vi "Basic ITC-IL.vi"(4 "Interval between messages (ms)":i16=10, 5 "ISOBUS address":T4=-1, 6 "error in (no error)":errorcluster, 7 "Device_Present?":bool[](array[boolean]), 8 "Ch_type_index":i32[](array[numeric]), 9 "Merc_ref_Array":T1[](array[typedef])) -> (0 "error out":errorcluster, 2 "Ch Info":T5(array[cluster]))   [LabVIEW 2013, in "Mercury iXX.lvlib"]
uses:
  Mercury iXX.lvlib
  Public/Libraries/Temperature/Signals/Read/Temperature (Read).vi
  Public/Libraries/Temperature.lvlib
  Public/Libraries/Level Meter/Signals/Read/Probe Level Helium (Read).vi
  Public/Libraries/Level Meter.lvlib
  Public/Libraries/Level Meter/Signals/Read/Probe Level Nitrogen (Read).vi
  Public/Controls/Comms Transport Layer.ctl
  Private/Controls/Query Dynamic Reference.ctl
  Public/Controls/Mercury Reference.ctl
  Public/Libraries/Heater/Signals/Read/Voltage (Read).vi
  Public/Libraries/Heater.lvlib
  Public/Libraries/Heater/Signals/Read/Current (Read).vi
  Public/Libraries/Heater/Signals/Read/Power (Read).vi
  Public/Libraries/Temperature/Signals/Read/Voltage (Read).vi
  Public/Libraries/Temperature/Signals/Read/Resistance (Read).vi
  Public/Libraries/Auxiliary/Signals/Read/Percent Open (Read).vi
  Public/Libraries/Auxiliary.lvlib
  Public/Libraries/Auxiliary/Signals/Read/Position (Read).vi
  Public/Libraries/Level Meter/Signals/Read/Probe Resistance Helium (Read).vi
  Public/Libraries/Level Meter/Signals/Read/Probe Frequency Nitrogen (Read).vi
  Public/Libraries/Pressure/Signals/Read/Pressure (Read).vi
  Public/Libraries/Pressure.lvlib
  Public/Libraries/Pressure/Signals/Read/Voltage (Read).vi
  Public/Libraries/Pressure/Signals/Read/Current (Read).vi
  Public/Libraries/Pressure/Signals/Read/Power (Read).vi
  Public/Controls/ISOBus Address.ctl
panel:
  in  "Tab Control":enum32{"Link Panel", "Front_Panel", "Error"}(tab)
  # "MB0\nMB1\nDB1\nDB2\nDB3\nDB4\nDB5\nDB6\nDB7\nDB8"
  # "Switch Controls"
  # "MercuryiTC-VI"
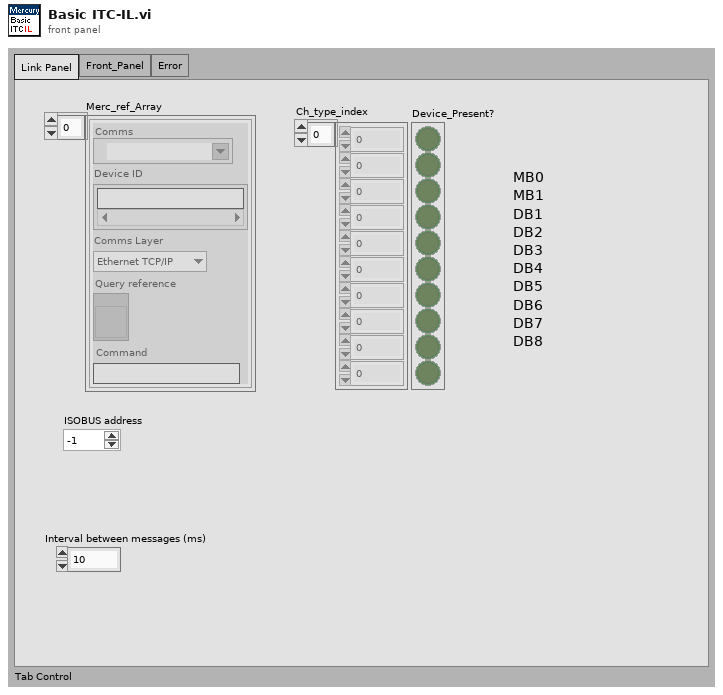
[diagram p1: front panel]
types:
  T1 = typedef "Mercury iXX.lvlib/Mercury Reference.ctl" = cluster{"Comms":refnum<visa-resource-name>, "Device ID":string[], "Comms Layer":T2, "Command":string, "Query reference":T3}
  T2 = typedef "Mercury iXX.lvlib/Comms Transport Layer.ctl" = enum16{"Ethernet TCP/IP", "USB", "ISOBus - RS-232", "GPIB"}
  T3 = typedef "Mercury iXX.lvlib/Query Dynamic Reference.ctl" = refnum<vi>
  T4 = typedef "Mercury iXX.lvlib/ISOBus Address.ctl" = i32
  T5 = cluster{"Data":string[], "Label":string[], "Units":string[], "Channel":string, "Type":string}[]
  T6 = cluster{"Data":string[], "Label":string[], "Units":string[], "Channel":string, "Type":string}
  T7 = typedef "Mercury iXX.lvlib/Unit String.ctl" = string
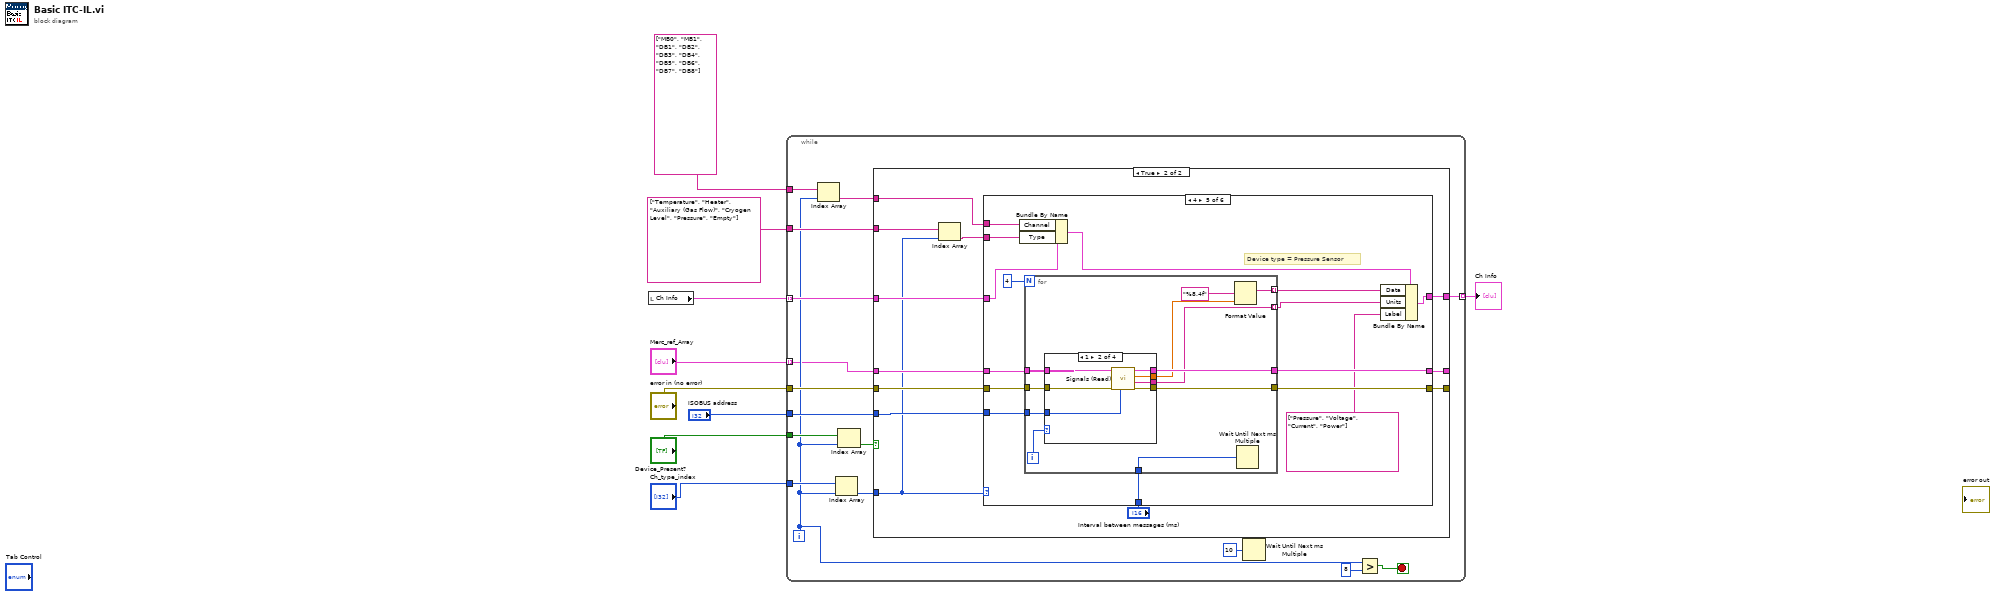
[diagram p0: block diagram]
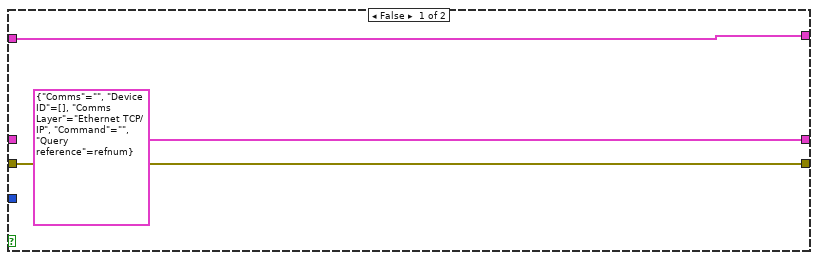
[diagram p2: hidden frame]
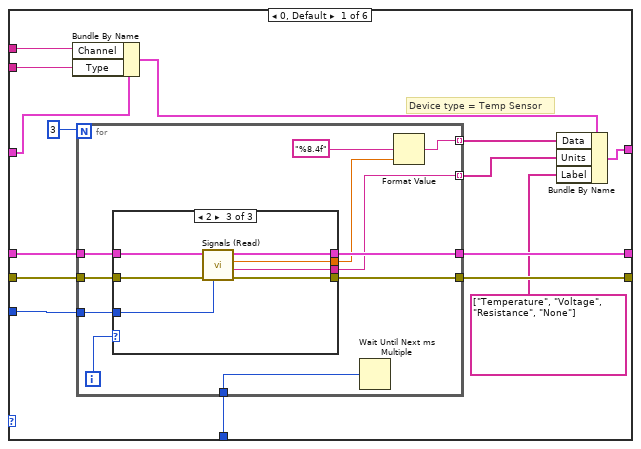
[diagram p3: hidden frame]
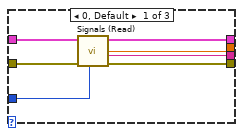
[diagram p4: hidden frame]
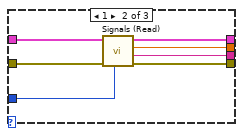
[diagram p5: hidden frame]
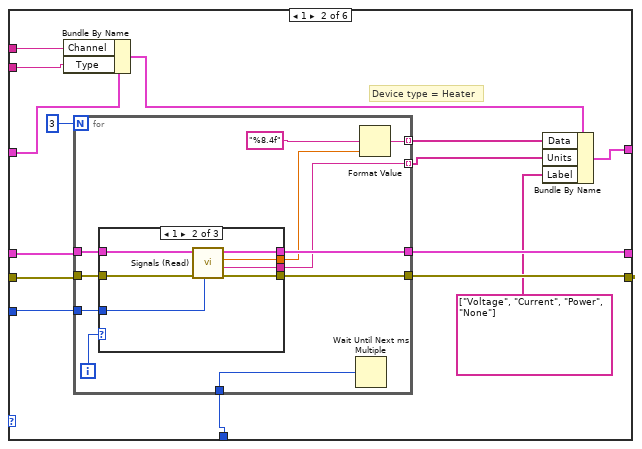
[diagram p6: hidden frame]
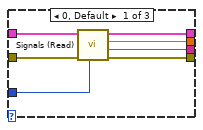
[diagram p7: hidden frame]
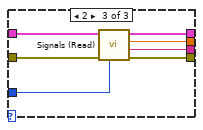
[diagram p8: hidden frame]
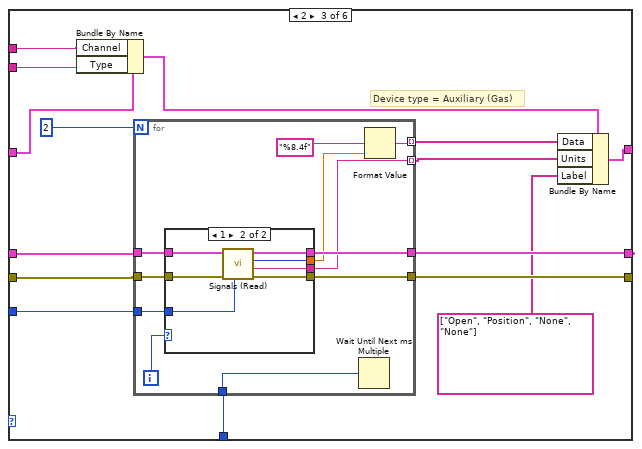
[diagram p9: hidden frame]
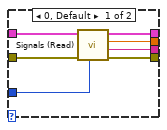
[diagram p10: hidden frame]
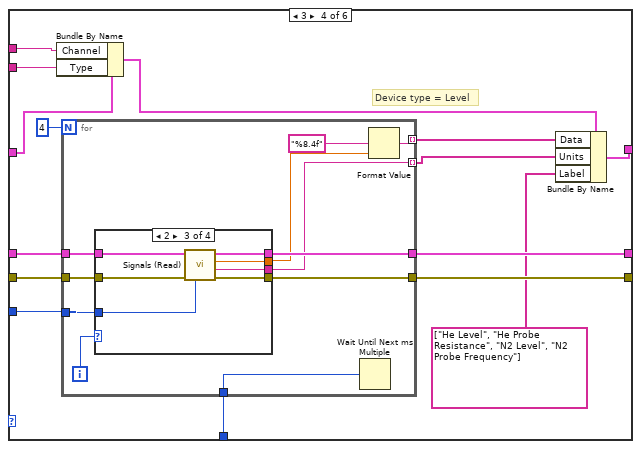
[diagram p11: hidden frame]
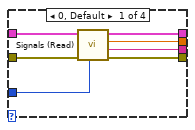
[diagram p12: hidden frame]
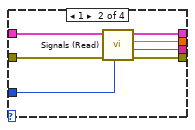
[diagram p13: hidden frame]
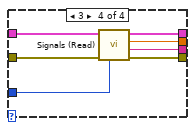
[diagram p14: hidden frame]
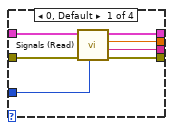
[diagram p15: hidden frame]
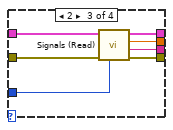
[diagram p16: hidden frame]
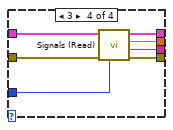
[diagram p17: hidden frame]
diagram:
  n1 = local read "Ch Info"() -> (w9:T5)
  n2 = while {
    tunnel: "Ch_type_index" -> [w25]
    tunnel: "Device_Present?" -> [w24]
    tunnel: "Merc_ref_Array" -> [w10] mode=indexing
    tunnel: "error in (no error)" -> [w21]
    tunnel: "ISOBUS address" -> [w20]
    tunnel: w9 -> [w19] mode=indexing
    tunnel: [w18] -> w3 mode=indexing
    tunnel: string[] ["Temperature", "Heater", "Auxiliary (Gas Flow)", "Cryogen Level", "Pressure", "Empty"] -> [w14]
    tunnel: string[] ["MB0", "MB1", "DB1", "DB2", "DB3", "DB4", "DB5", "DB6", "DB7", "DB8"] -> [w13]
    i -> [w12]
    stop <- w17 stop-if-true
    n3 = Index Array(array=w13, index=w12) -> (element=w11:string)
    n4 = Index Array(array=w25, index=w12) -> (element=w22:i32)
    n5 = Index Array(array=w24, index=w12) -> (element=w23:bool)
    n6 = case shown="True" w23 {
      tunnel: w10 -> [_ w40]
      tunnel: w22 -> [_ w31]
      tunnel: w21 -> [w27 w39]
      tunnel: w20 -> [_ w38]
      tunnel: [w27 w37] -> _
      tunnel: [T1 {"Comms"="", "Device ID"=[], "Comms Layer"=enum."Ethernet TCP/IP", "Command"="", "Query reference"=refnum} ("MB1.T1_Ref") w36] -> _
      tunnel: w19 -> [w26 w34]
      tunnel: [w26 w33] -> w18
      tunnel: w14 -> [_ w32]
      tunnel: w11 -> [_ w29]
      frame False {
      }
      frame True {
        n7 = Index Array(array=w32, index=w31) -> (element=w30:string)
        n8 = case shown="4" w31 {
          tunnel: w40 -> [w55 w102 w149 w189 w243 w285]
          tunnel: w39 -> [w54 w101 w148 w188 w242 w284]
          tunnel: w38 -> [w52 w100 w147 w187 w241 _]
          tunnel: [w51 w98 w145 w185 w239 w285] -> w36
          tunnel: [w50 w97 w144 w184 w238 w284] -> w37
          tunnel: "Interval between messages (ms)" -> [w53 w99 w146 w186 w240 _]
          tunnel: w34 -> [w41 w89 w138 w176 w230 w283]
          tunnel: [w48 w95 w142 w182 w236 w283] -> w33
          tunnel: w30 -> [w44 w90 w136 w177 w231 _]
          tunnel: w29 -> [w43 w91 w137 w178 w232 _]
          frame 0, Default {
            # "Device type = Temp Sensor"
            n9 = Bundle By Name(cluster=w41, "Channel"=w43, "Type"=w44) -> (w42:T6)
            n10 = for {
              N: 3 -> [_]
              tunnel: w55 -> [w65]
              tunnel: w54 -> [w64]
              tunnel: w53 -> [w63]
              tunnel: w52 -> [w62]
              tunnel: [w61] -> w51
              tunnel: [w60] -> w50
              tunnel: [w58] -> w47 mode=indexing
              tunnel: [w56] -> w45 mode=indexing
              i -> [w66]
              n11 = case shown="2" w66 {
                tunnel: w65 -> [w73 w80 w86]
                tunnel: w64 -> [w72 w79 w85]
                tunnel: w62 -> [w71 w78 w87]
                tunnel: [w70 w77 w84] -> w61
                tunnel: [w69 w76 w83] -> w60
                tunnel: [w68 w75 w82] -> w59
                tunnel: [w67 w74 w81] -> w56
                frame 0, Default {
                  n12 = call-poly "Signals (Read).vi"("ISOBUS address"=w71, "error in"=w72, "Mercury Reference In"=w73) -> ("error out"=w69:errorcluster, "Unit"=w67:T7, "Temperature"=w68:dbl, "Mercury Reference Out"=w70:T1)  [unwired: 4 in, 1 out]
                }
                frame 1 {
                  n13 = call-poly "Signals (Read).vi"("ISOBUS address"=w78, "error in"=w79, "Mercury Reference In"=w80) -> ("error out"=w76:errorcluster, "Unit"=w74:T7, "Voltage"=w75:dbl, "Mercury Reference Out"=w77:T1)  [unwired: 4 in, 1 out]
                }
                frame 2 {
                  n14 = call-poly "Signals (Read).vi"("ISOBUS address"=w87, "error in"=w85, "Mercury Reference In"=w86) -> ("error out"=w83:errorcluster, "Unit"=w81:T7, "Resistance"=w82:dbl, "Mercury Reference Out"=w84:T1)  [unwired: 4 in, 1 out]
                }
              }
              n15 = Wait Until Next ms Multiple(millisecond multiple=w63) -> ()  [unwired: 1 out]
              n16 = Format Value(format string="%8.4f", value (0)=w59) -> (output string=w58:string)  [unwired: 1 in]
            }
            n17 = Bundle By Name(cluster=w42, "Data"=w47, "Units"=w45, "Label"=string[] ["Temperature", "Voltage", "Resistance", "None"]) -> (w48:T6)
          }
          frame 1 {
            # "Device type = Heater"
            n18 = Bundle By Name(cluster=w89, "Channel"=w91, "Type"=w90) -> (w88:T6)
            n19 = for {
              N: 3 -> [_]
              tunnel: w102 -> [w112]
              tunnel: w101 -> [w111]
              tunnel: w99 -> [w110]
              tunnel: w100 -> [w109]
              tunnel: [w108] -> w98
              tunnel: [w107] -> w97
              tunnel: [w105] -> w94 mode=indexing
              tunnel: [w103] -> w92 mode=indexing
              i -> [w113]
              n20 = case shown="1" w113 {
                tunnel: w112 -> [w120 w127 w133]
                tunnel: w111 -> [w119 w126 w132]
                tunnel: w109 -> [w118 w125 w134]
                tunnel: [w117 w124 w131] -> w108
                tunnel: [w116 w123 w130] -> w107
                tunnel: [w115 w122 w129] -> w106
                tunnel: [w114 w121 w128] -> w103
                frame 0, Default {
                  n21 = call-poly "Signals (Read).vi"("ISOBUS address"=w118, "error in"=w119, "Mercury Reference In"=w120) -> ("error out"=w116:errorcluster, "Unit"=w114:T7, "Voltage"=w115:dbl, "Mercury Reference Out"=w117:T1)  [unwired: 4 in, 1 out]
                }
                frame 1 {
                  n22 = call-poly "Signals (Read).vi"("ISOBUS address"=w125, "error in"=w126, "Mercury Reference In"=w127) -> ("error out"=w123:errorcluster, "Unit"=w121:T7, "Current"=w122:dbl, "Mercury Reference Out"=w124:T1)  [unwired: 4 in, 1 out]
                }
                frame 2 {
                  n23 = call-poly "Signals (Read).vi"("ISOBUS address"=w134, "error in"=w132, "Mercury Reference In"=w133) -> ("error out"=w130:errorcluster, "Unit"=w128:T7, "Power"=w129:dbl, "Mercury Reference Out"=w131:T1)  [unwired: 4 in, 1 out]
                }
              }
              n24 = Wait Until Next ms Multiple(millisecond multiple=w110) -> ()  [unwired: 1 out]
              n25 = Format Value(format string="%8.4f", value (0)=w106) -> (output string=w105:string)  [unwired: 1 in]
            }
            n26 = Bundle By Name(cluster=w88, "Data"=w94, "Units"=w92, "Label"=string[] ["Voltage", "Current", "Power", "None"]) -> (w95:T6)
          }
          frame 2 {
            # "Device type = Auxiliary (Gas)"
            n27 = Bundle By Name(cluster=w138, "Channel"=w137, "Type"=w136) -> (w135:T6)
            n28 = for {
              N: 2 -> [_]
              tunnel: w149 -> [w159]
              tunnel: w148 -> [w158]
              tunnel: w146 -> [w157]
              tunnel: w147 -> [w156]
              tunnel: [w155] -> w145
              tunnel: [w154] -> w144
              tunnel: [w151] -> w141 mode=indexing
              tunnel: [w150] -> w139 mode=indexing
              i -> [w160]
              n29 = case shown="1" w160 {
                tunnel: w159 -> [w167 w174]
                tunnel: w158 -> [w166 w173]
                tunnel: w156 -> [w165 w172]
                tunnel: [w164 w171] -> w155
                tunnel: [w163 w170] -> w154
                tunnel: [w162 w169] -> w152
                tunnel: [w161 w168] -> w150
                frame 0, Default {
                  n30 = call-poly "Signals (Read).vi"("ISOBUS address"=w165, "error in"=w166, "Mercury Reference In"=w167) -> ("error out"=w163:errorcluster, "Unit"=w161:T7, "% Open"=w162:dbl, "Mercury Reference Out"=w164:T1)  [unwired: 4 in, 1 out]
                }
                frame 1 {
                  n31 = call-poly "Signals (Read).vi"("ISOBUS address"=w172, "error in"=w173, "Mercury Reference In"=w174) -> ("error out"=w170:errorcluster, "Unit"=w168:T7, "Position"=w169:u32, "Mercury Reference Out"=w171:T1)  [unwired: 4 in, 1 out]
                }
              }
              n32 = Wait Until Next ms Multiple(millisecond multiple=w157) -> ()  [unwired: 1 out]
              n33 = Format Value(format string="%8.4f", value (0)=w152) -> (output string=w151:string)  [unwired: 1 in]
            }
            n34 = Bundle By Name(cluster=w135, "Data"=w141, "Units"=w139, "Label"=string[] ["Open", "Position", "None", "None"]) -> (w142:T6)
          }
          frame 3 {
            # "Device type = Level"
            n35 = Bundle By Name(cluster=w176, "Channel"=w178, "Type"=w177) -> (w175:T6)
            n36 = for {
              N: 4 -> [_]
              tunnel: w189 -> [w199]
              tunnel: w188 -> [w198]
              tunnel: w186 -> [w197]
              tunnel: w187 -> [w196]
              tunnel: [w195] -> w185
              tunnel: [w194] -> w184
              tunnel: [w191] -> w181 mode=indexing
              tunnel: [w190] -> w179 mode=indexing
              i -> [w200]
              n37 = case shown="2" w200 {
                tunnel: w199 -> [w207 w214 w220 w227]
                tunnel: w198 -> [w206 w213 w219 w226]
                tunnel: w196 -> [w205 w212 w221 w228]
                tunnel: [w204 w211 w218 w225] -> w195
                tunnel: [w203 w210 w217 w224] -> w194
                tunnel: [w202 w209 w216 w223] -> w192
                tunnel: [w201 w208 w215 w222] -> w190
                frame 0, Default {
                  n38 = call-poly "Signals (Read).vi"("ISOBUS address"=w205, "error in"=w206, "Mercury Reference In"=w207) -> ("error out"=w203:errorcluster, "Unit"=w201:T7, "Level"=w202:dbl, "Mercury Reference Out"=w204:T1)  [unwired: 4 in, 1 out]
                }
                frame 1 {
                  n39 = call-poly "Signals (Read).vi"("ISOBUS address"=w212, "error in"=w213, "Mercury Reference In"=w214) -> ("error out"=w210:errorcluster, "Unit"=w208:T7, "Resistance"=w209:dbl, "Mercury Reference Out"=w211:T1)  [unwired: 4 in, 1 out]
                }
                frame 2 {
                  n40 = call-poly "Signals (Read).vi"("ISOBUS address"=w221, "error in"=w219, "Mercury Reference In"=w220) -> ("error out"=w217:errorcluster, "Unit"=w215:T7, "Level"=w216:dbl, "Mercury Reference Out"=w218:T1)  [unwired: 4 in, 1 out]
                }
                frame 3 {
                  n41 = call-poly "Signals (Read).vi"("ISOBUS address"=w228, "error in"=w226, "Mercury Reference In"=w227) -> ("error out"=w224:errorcluster, "Unit"=w222:T7, "Freq"=w223:dbl, "Mercury Reference Out"=w225:T1)  [unwired: 4 in, 1 out]
                }
              }
              n42 = Wait Until Next ms Multiple(millisecond multiple=w197) -> ()  [unwired: 1 out]
              n43 = Format Value(format string="%8.4f", value (0)=w192) -> (output string=w191:string)  [unwired: 1 in]
            }
            n44 = Bundle By Name(cluster=w175, "Data"=w181, "Units"=w179, "Label"=string[] ["He Level", "He Probe Resistance", "N2 Level", "N2 Probe Frequency"]) -> (w182:T6)
          }
          frame 4 {
            # "Device type = Pressure Sensor"
            n45 = Bundle By Name(cluster=w230, "Channel"=w232, "Type"=w231) -> (w229:T6)
            n46 = for {
              N: 4 -> [_]
              tunnel: w243 -> [w253]
              tunnel: w242 -> [w252]
              tunnel: w240 -> [w251]
              tunnel: w241 -> [w250]
              tunnel: [w249] -> w239
              tunnel: [w248] -> w238
              tunnel: [w245] -> w235 mode=indexing
              tunnel: [w244] -> w233 mode=indexing
              i -> [w254]
              n47 = case shown="1" w254 {
                tunnel: w253 -> [w261 w268 w274 w281]
                tunnel: w252 -> [w260 w267 w273 w280]
                tunnel: w250 -> [w259 w266 w275 w282]
                tunnel: [w258 w265 w272 w279] -> w249
                tunnel: [w257 w264 w271 w278] -> w248
                tunnel: [w256 w263 w270 w277] -> w247
                tunnel: [w255 w262 w269 w276] -> w244
                frame 0, Default {
                  n48 = call-poly "Signals (Read).vi"("ISOBUS address"=w259, "error in"=w260, "Mercury Reference In"=w261) -> ("error out"=w257:errorcluster, "Unit"=w255:T7, "Temperature"=w256:dbl, "Mercury Reference Out"=w258:T1)  [unwired: 4 in, 1 out]
                }
                frame 1 {
                  n49 = call-poly "Signals (Read).vi"("ISOBUS address"=w266, "error in"=w267, "Mercury Reference In"=w268) -> ("error out"=w264:errorcluster, "Unit"=w262:T7, "Voltage"=w263:dbl, "Mercury Reference Out"=w265:T1)  [unwired: 4 in, 1 out]
                }
                frame 2 {
                  n50 = call-poly "Signals (Read).vi"("ISOBUS address"=w275, "error in"=w273, "Mercury Reference In"=w274) -> ("error out"=w271:errorcluster, "Unit"=w269:T7, "Current"=w270:dbl, "Mercury Reference Out"=w272:T1)  [unwired: 4 in, 1 out]
                }
                frame 3 {
                  n51 = call-poly "Signals (Read).vi"("ISOBUS address"=w282, "error in"=w280, "Mercury Reference In"=w281) -> ("error out"=w278:errorcluster, "Unit"=w276:T7, "Power"=w277:dbl, "Mercury Reference Out"=w279:T1)  [unwired: 4 in, 1 out]
                }
              }
              n52 = Format Value(format string="%8.4f", value (0)=w247) -> (output string=w245:string)  [unwired: 1 in]
              n53 = Wait Until Next ms Multiple(millisecond multiple=w251) -> ()  [unwired: 1 out]
            }
            n54 = Bundle By Name(cluster=w229, "Data"=w235, "Units"=w233, "Label"=string[] ["Pressure", "Voltage", "Current", "Power"]) -> (w236:T6)
          }
          frame 5 {
            # "Device type = None"
          }
        }
      }
    }
    n55 = Wait Until Next ms Multiple(millisecond multiple=u32 10) -> ()  [unwired: 1 out]
    n56 = Greater?(x=w12, y=8) -> (0:w17:bool)
  }
  "Ch Info" <- w3
